vi "getTimeoutActuatorIds.vi"(11 "ILCCommunications in":refnum<class "ILCCommunications.lvclass">) -> (2 "TimeoutActuatorIds":i32[](array[numeric]), 3 "ILCCommunications out":refnum<class "ILCCommunications.lvclass">)   [LabVIEW 2016, in "ILCCommunications.lvclass"]
uses:
  ILCCommunications.lvclass
  ILCCommunications.lvclass/ILCCommunications.ctl
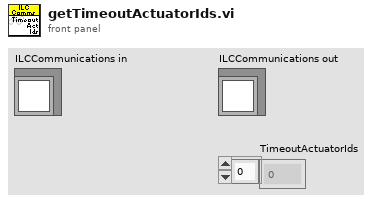
[diagram p1: front panel]
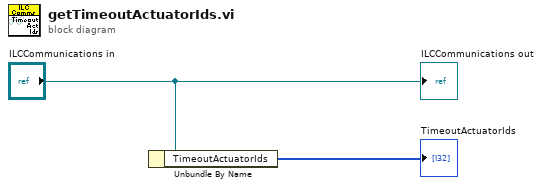
[diagram p0: block diagram]
diagram:
  n1 = Unbundle By Name("ILCCommunications in") -> ("TimeoutActuatorIds"=→"TimeoutActuatorIds":i32[])
  "ILCCommunications out" <- "ILCCommunications in"
